vi "Add DIO Card From Table.vi"(8 "error in (no error)":errorcluster, 10 "Card Position":T1 {"Slot #" max=15}, 11 "Node Ptr":u64 format="%.0x") -> (0 "error out":errorcluster)   [LabVIEW 2014, in "SLSC configuration System Explorer.lvlib"]
uses:
  SLSC configuration System Explorer.lvlib
  Type Defs/Card Position.ctl
  Example/SPI Utility/Slot #.ctl
  Shared/Constants.vi
  <vilib>/NI Veristand/Custom Device API/Set Item Property (U16).vi
  <vilib>/NI Veristand/Custom Device API/Custom Device API.lvlib
  Shared/SLSC configuration Shared.lvlib
  <vilib>/NI Veristand/Custom Device Tools/Custom Device Utility Library/Custom Device Utility Library.lvlib
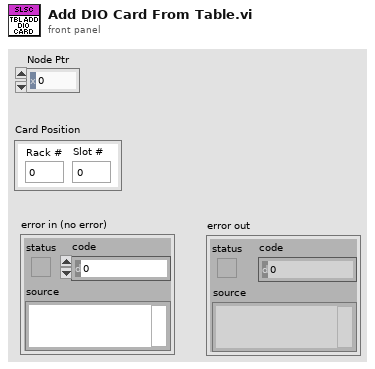
[diagram p1: front panel]
types:
  T1 = typedef "SLSC configuration Shared.lvlib/Card Position.ctl" = cluster{"Rack #":u8, "Slot #":T2}
  T2 = typedef "SLSC configuration Shared.lvlib/Slot #.ctl" = u8
  T3 = typedef "Custom Device API.lvlib/Custom Device Item Ref.ctl" = u64
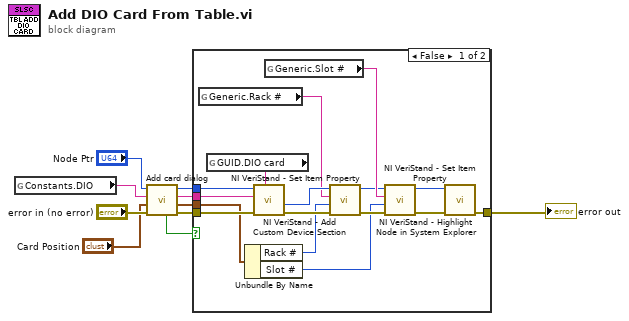
[diagram p0: block diagram]
diagram:
  n1 = global read "Constants.vi" "Constants.DIO"() -> (w4:string)
  n2 = call "Add card dialog.vi"("error in (no error)"="error in (no error)", "Card Position"="Card Position", "Card Type in"=w4, "Node Ptr"="Node Ptr") -> ("error out"=w8:errorcluster, "Card Position out"=w5:cluster{"Rack #":u8, "Slot #":T2}, "Name out"=w7:string, "Node Ptr out"=w6:u64, "Cancelled?"=w1:bool)  [unwired: 3 in]
  n3 = case shown="False" w1 {
    tunnel: w8 -> [w24 w27]
    tunnel: w7 -> [w23 _]
    tunnel: w6 -> [w22 _]
    tunnel: w5 -> [w19 _]
    tunnel: [w12 w27] -> w3
    frame False {
      n4 = global read "Constants.vi" "Generic.Rack #"() -> (w20:string)
      n5 = global read "Constants.vi" "GUID.DIO card"() -> (w25:string)
      n6 = Unbundle By Name(w19) -> ("Rack #"=w18:u8, "Slot #"=w14:T2)
      n7 = call <vilib>:"NI VeriStand - Add Custom Device Section.vi"("GUID (Default Section)"=w25, "error in (no error)"=w24, "Section Name"=w23, "Parent Ref in"=w22) -> ("error out"=w26:errorcluster, "Section Ptr"=w21:T3)  [unwired: 4 in, 2 out]
      n8 = global read "Constants.vi" "Generic.Slot #"() -> (w17:string)
      n9 = call-poly <vilib>:"NI VeriStand - Set Item Property.vi"("error in (no error)"=w26, "Value"=w18, "Property Name"=w20, "Item Ref in"=w21) -> ("error out"=w16:errorcluster, "Item Ref out"=w15:T3)  [unwired: 5 in, 1 out]
      n10 = call-poly <vilib>:"NI VeriStand - Set Item Property.vi"("error in (no error)"=w16, "Value"=w14, "Property Name"=w17, "Item Ref in"=w15) -> ("error out"=w13:errorcluster, "Item Ref out"=w11:T3)  [unwired: 5 in, 1 out]
      n11 = call <vilib>:"NI VeriStand - Highlight Node in System Explorer.vi"("error in (no error)"=w13, "Item Ref in"=w11) -> ("error out"=w12:errorcluster)  [unwired: 8 in, 1 out]
    }
    frame True {
    }
  }
  "error out" <- w3
